vi "pbr-builder.vi"(9 "FLOW in":T3[](array[typedef]), 11 "PBR FLOW in":T2(array[cluster])) -> (1 "PBR FLOW OUT":T2(array[cluster])=[{"Operation"=enum."DELAY SEC", "Param"="5", "uid"=""}, {"Operation"=enum."SENSE", "Param"="5", "uid"=""}, {"Operation"=enum."SENSE", "Param"="a1 > 1.23", "uid"=""}, {"Operation"=enum."SET OUTPUT", "Param"="o1 ON 44", "uid"=""}, {"Operation"=enum."PROC START", "Param"="PROC1", "uid"=""}, {"Operation"=enum."SET OUTPUT", "Param"="PROC1", "uid"=""}], 2 "Err":errorcluster, 3 "FLOW out":T3[](array[typedef]))   [LabVIEW 2024]
uses:
  controls/UiStepBuilder.ctl
  controls/type.step-builder.ctl
  controls/pbr-func-def.ctl
  controls/UiDeviceSensorParams.ctl
  controls/UiDeviceSensorEquality.ctl
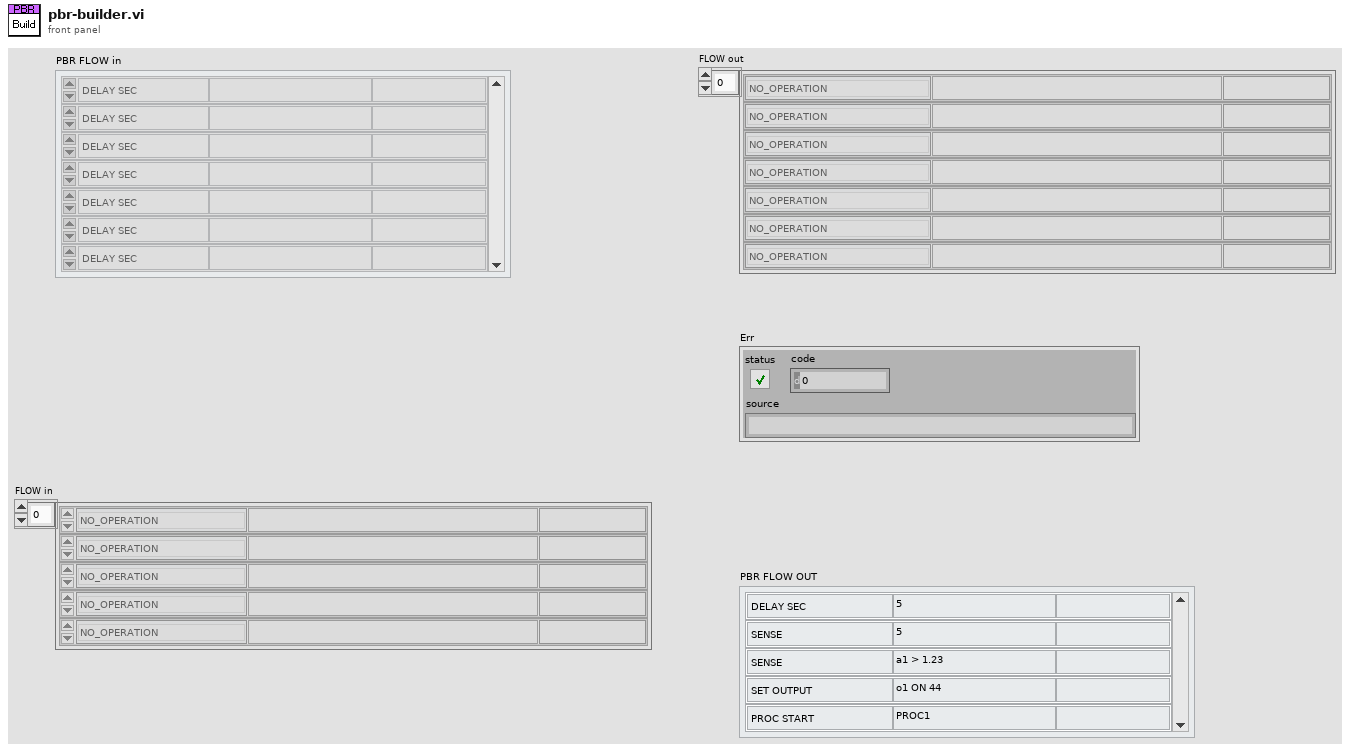
[diagram p1: front panel]
types:
  T1 = typedef "pbr-func-def.ctl" = enum16{"DELAY SEC", "SCHEDULE DAILY", "SENSE", "PROC START", "SET OUTPUT", "FINISH", "JUMP"}
  T2 = cluster{"Operation":T1, "Param":string, "uid":string}[]
  T3 = typedef "UiStepBuilder.ctl" = cluster{"Step Function":T4, "ParamString":string, "Step Label":string}
  T4 = typedef "type.step-builder.ctl" = enum16{"NO_OPERATION", "DELAY-JUMP", "DELAY", "JUMP", "COMPLETE", "SCHEDULER", "SCHEDULER_DAILY", "IRR-CHECK", "UNIT-CHECK", "UNIT-SAMPLE", "UNIT-DOSE", "LOG-REPORT", "LOG-MESSAGE", "IO-READ", "IO-READ-MANY", "IO-WRITE", "IO-COMPARE-OUT", "IO-COMPARE-IN", "PROC-START", "PROC-STOP", "PROC-LOAD", "PROC-IS-COMPLETED", "RECORD-MOVE", "GET-RH", "GET-UV", "GET-WD", "GET-WS", "OCS-CHECK", "OCS-RECORD"}
  T5 = typedef "UiDeviceSensorParams.ctl" = cluster{"Input":string, "Comparison":T6, "Setpoint":dbl}
  T6 = typedef "UiDeviceSensorEquality.ctl" = string
  T7 = cluster{"Operation":T1, "Param":string, "Label":string}
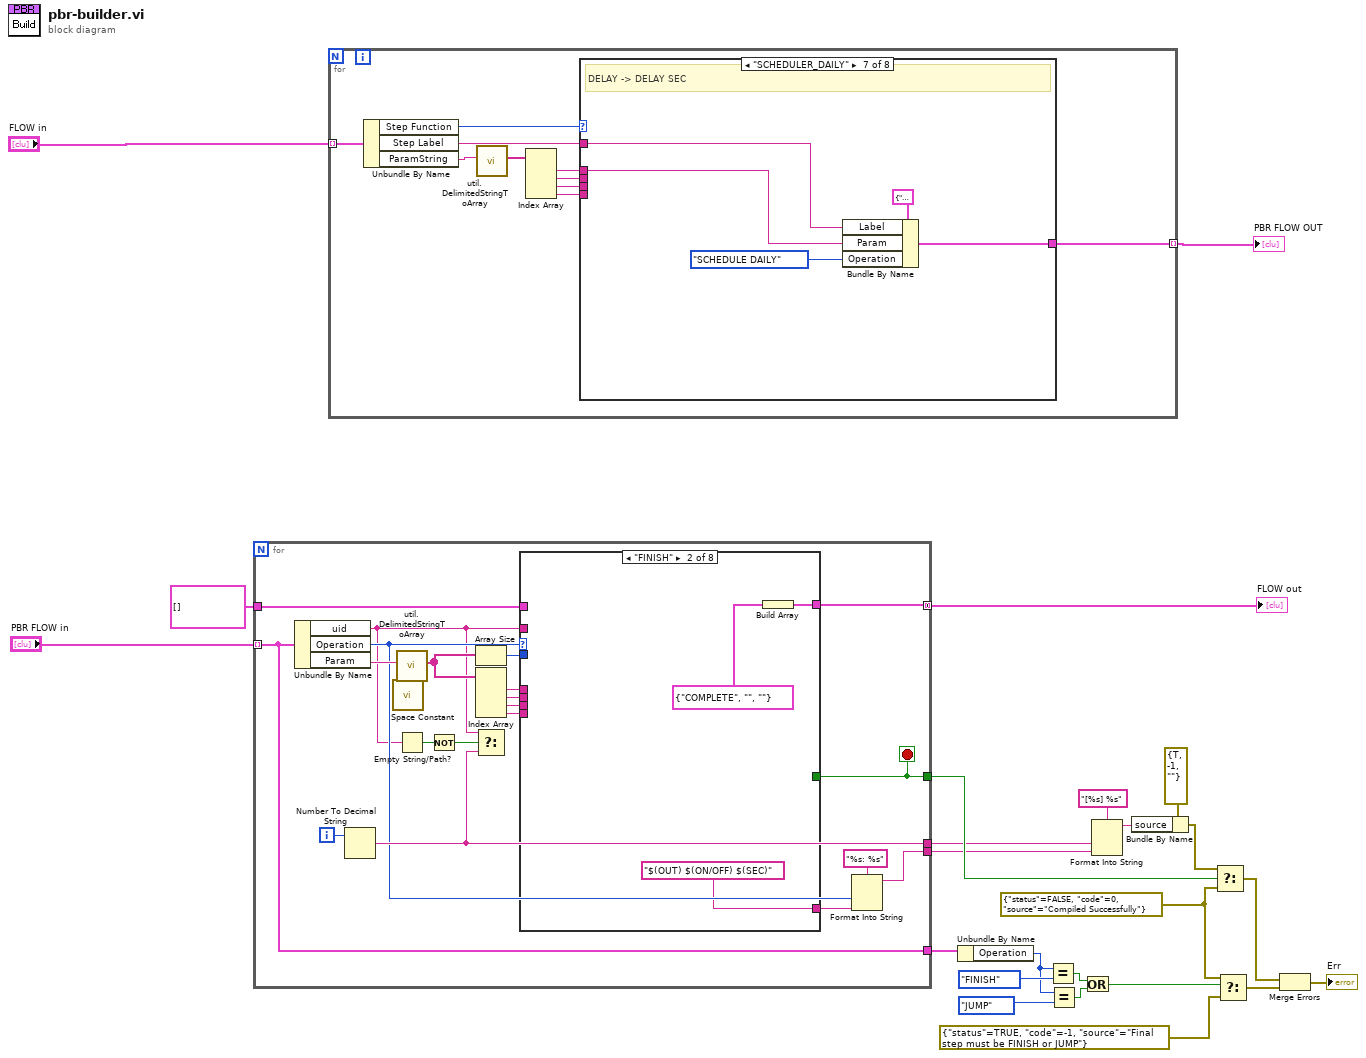
[diagram p0: block diagram]
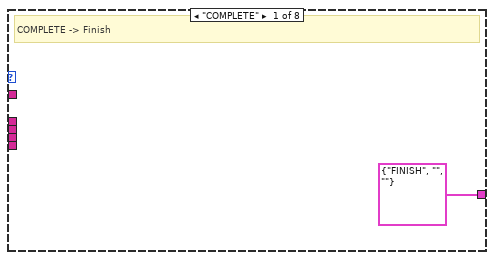
[diagram p2: hidden frame]
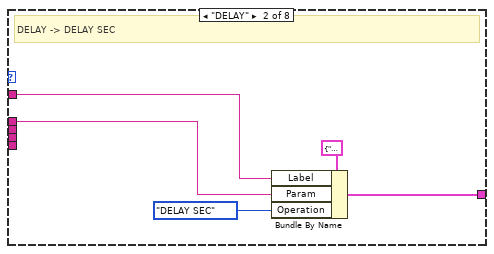
[diagram p3: hidden frame]
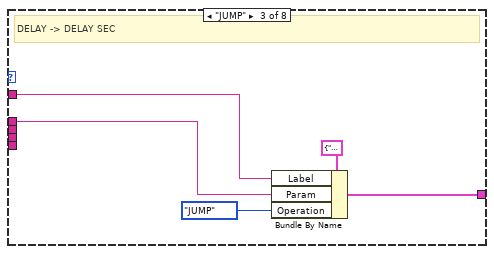
[diagram p4: hidden frame]
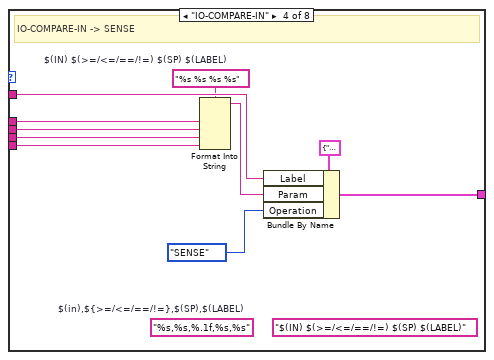
[diagram p5: hidden frame]
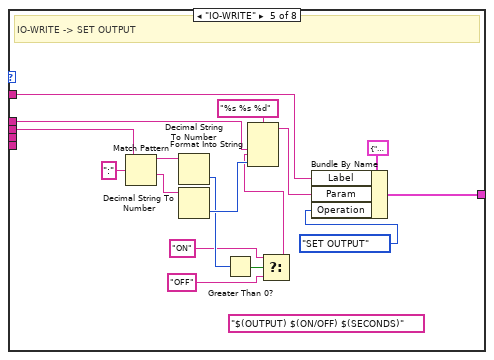
[diagram p6: hidden frame]
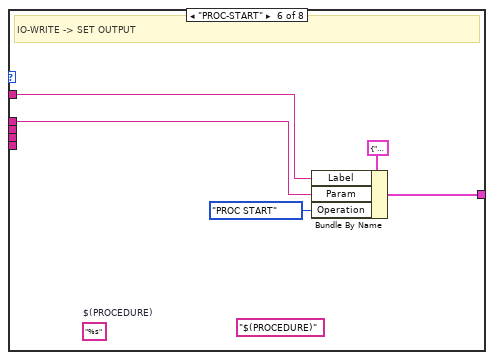
[diagram p7: hidden frame]
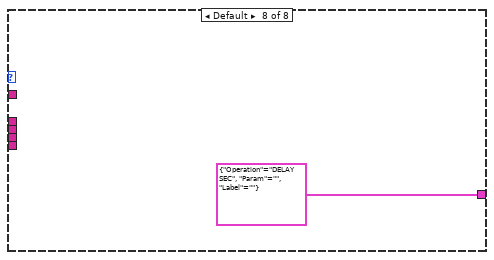
[diagram p8: hidden frame]
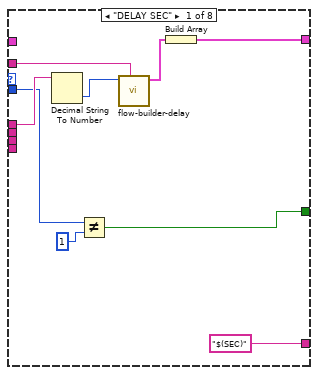
[diagram p9: hidden frame]
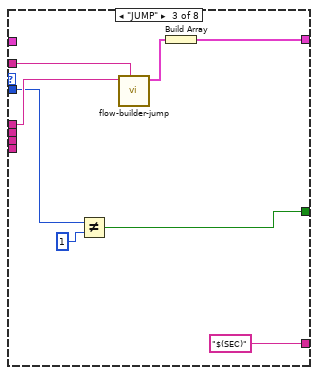
[diagram p10: hidden frame]
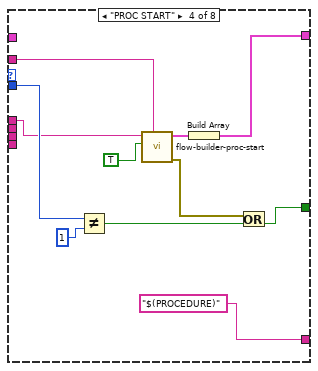
[diagram p11: hidden frame]
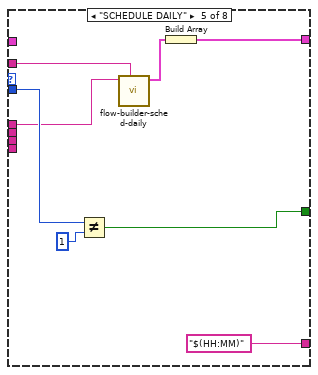
[diagram p12: hidden frame]
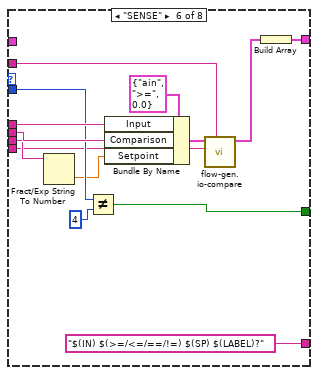
[diagram p13: hidden frame]
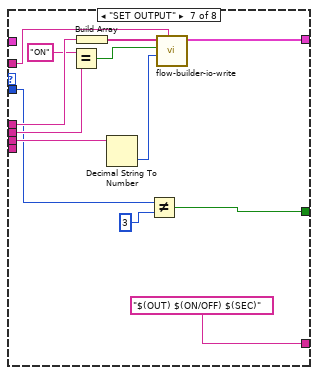
[diagram p14: hidden frame]
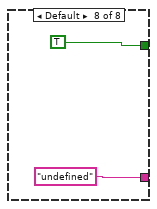
[diagram p15: hidden frame]
diagram:
  w2 = errorcluster {"status"=FALSE, "code"=0, "source"="Compiled Successfully"} ("error constant")
  n1 = for {
    tunnel: "PBR FLOW in" -> [w26] mode=indexing
    tunnel: [w45] -> w13 mode=concatenating
    tunnel: T3[] [] ("UiBuildSteps") -> [w42]
    tunnel: [w35] -> w22
    tunnel: [w34] -> w20
    tunnel: [w28] -> w16
    tunnel: [w26] -> w12
    i -> [w38]
    stop <- w35 stop-if-true
    n2 = Unbundle By Name(w26) -> ("uid"=w25:string, "Operation"=w30:T1, "Param"=w44:string)
    n3 = Number To Decimal String(number=w38) -> (decimal integer string=w34:string)  [unwired: 1 in]
    n4 = call <vilib>:"Space Constant.vi"() -> ("String"=w43:string)
    n5 = call "util.DelimitedStringToArray.vi"("delimiter (,)"=w43, "delimitaed string"=w44) -> ("array out"=w33:string[])  [unwired: 9 in]
    n6 = Empty String/Path?(string/path=w25) -> (empty?=w37:bool)
    n7 = Not(x=w37) -> (.not. x?=w36:bool)
    n8 = Array Size(array=w33) -> (size(s)=w32:i32)
    n9 = Index Array(array=w33) -> (element #1=w41:string, element #2=w40:string, element #3=w39:string, element #4=w27:string)  [unwired: 4 in]
    n10 = Select(t=w25, s=w36, f=w34) -> ()  [unwired: 1 out]
    n11 = case shown="\"FINISH\"" w30 {
      tunnel: w42 -> [_ _ _ _ _ _ _ _]
      tunnel: [w53 w55 w64 w76 w83 w95 w111 _] -> w45
      tunnel: [w47 _ w59 w67 w79 w90 w101 TRUE] -> w35
      tunnel: w41 -> [w52 _ w63 w69 w77 w98 w110 _]
      tunnel: w40 -> [_ _ _ _ _ w97 w108 _]
      tunnel: w25 -> [w50 _ w62 w70 w82 w94 w99 _]
      tunnel: w39 -> [_ _ _ _ _ w96 w104 _]
      tunnel: w32 -> [w48 _ w60 w74 w80 w91 w103 _]
      tunnel: ["$(SEC)" ("y") "$(OUT) $(ON/OFF) $(SEC)" ("y") "$(SEC)" ("y") "$(PROCEDURE)" ("y") "$(HH:MM)" ("y") "$(IN) $(>=/<=/==/!=) $(SP) $(LABEL)?" ("y") "$(OUT) $(ON/OFF) $(SEC)" ("y") "undefined" ("format string")] -> w29
      tunnel: w27 -> [_ _ _ _ _ w85 _ _]
      frame "DELAY SEC" {
        n12 = Decimal String To Number(string=w52) -> (number=w51:i32)  [unwired: 2 in, 1 out]
        n13 = Not Equal?(x=w48, y=1) -> (x != y?=w47:bool)
        n14 = call "flow-builder-delay.vi"("Step Label"=w50, "Delay [s]"=w51) -> ("Step Element"=w54:T3)  [unwired: 9 in]
        n15 = Build Array(w54) -> (w53:T3[])
      }
      frame "FINISH" {
        n16 = Build Array(T3 {"Step Function"=enum."COMPLETE", "ParamString"="", "Step Label"=""} ("FlowModeConstant 2")) -> (w55:T3[])
      }
      frame "JUMP" {
        n17 = Not Equal?(x=w60, y=1) -> (x != y?=w59:bool)
        n18 = call "flow-builder-jump.vi"("Step Label"=w62, "StepPtr"=w63) -> ("Step Element"=w65:T3)  [unwired: 9 in]
        n19 = Build Array(w65) -> (w64:T3[])
      }
      frame "PROC START" {
        n20 = Not Equal?(x=w74, y=1) -> (x != y?=w73:bool)
        n21 = call "flow-builder-proc-start.vi"("Step Label"=w70, "Start(T) / Stop(F)"=TRUE, "Proc Name"=w69) -> ("Error"=w66:errorcluster, "Step Element"=w71:T3)  [unwired: 7 in]
        n22 = Build Array(w71) -> (w76:T3[])
        n23 = Or(x=w66, y=w73) -> (x .or. y?=w67:bool)
      }
      frame "SCHEDULE DAILY" {
        n24 = Not Equal?(x=w80, y=1) -> (x != y?=w79:bool)
        n25 = call "flow-builder-sched-daily.vi"("Step Label"=w82, "time (HH:MM)"=w77) -> ("Step Element"=w84:T3)  [unwired: 9 in]
        n26 = Build Array(w84) -> (w83:T3[])
      }
      frame "SENSE" {
        n27 = Fract/Exp String To Number(string=w96) -> (number=w89:dbl)  [unwired: 3 in, 1 out]
        n28 = Not Equal?(x=w91, y=4) -> (x != y?=w90:bool)
        n29 = Bundle By Name(cluster=T5 {"Input"="ain", "Comparison"=">=", "Setpoint"=0.0} ("Device Sensor Params"), "Input"=w98, "Comparison"=w97, "Setpoint"=w89) -> (w87:T5)
        n30 = call "flow-gen.io-compare.vi"("Step Label"=w94, "stepPointer (False Cond.)"=w85, "Device Sensor Params"=w87) -> ("Step out"=w86:T3)  [unwired: 8 in]
        n31 = Build Array(w86) -> (w95:T3[])
      }
      frame "SET OUTPUT" {
        n32 = Equal?(x=w108, y="ON") -> (x = y?=w106:bool)
        n33 = Build Array(w110) -> (w109:string[])
        n34 = Decimal String To Number(string=w104) -> (number=w105:i32)  [unwired: 2 in, 1 out]
        n35 = Not Equal?(x=w103, y=3) -> (x != y?=w101:bool)
        n36 = call "flow-builder-io-write.vi"("Step Name"=w99, "Digital Timeout"=w105, "Value in"=w106, "Dout+AUX"=w109) -> ("Flow out"=w111:T3[])  [unwired: 7 in]
      }
      frame Default {
      }
    }
    n37 = Format Into String(format string="%s: %s", w30, w29) -> (resulting string=w28:string)  [unwired: 2 in, 1 out]
  }
  "FLOW out" <- w13
  n38 = for {
    tunnel: "FLOW in" -> [w123] mode=indexing
    tunnel: [w121] -> w15 mode=indexing
    n39 = Unbundle By Name(w123) -> ("Step Function"=w122:T4, "Step Label"=w120:string, "ParamString"=w119:string)
    n40 = call "util.DelimitedStringToArray.vi"("delimitaed string"=w119) -> ("array out"=w118:string[])  [unwired: 10 in]
    n41 = Index Array(array=w118) -> (element #1=w117:string, element #2=w116:string, element #3=w115:string, element #4=w114:string)  [unwired: 4 in]
    n42 = case shown="\"SCHEDULER_DAILY\"" w122 {
      tunnel: [T7 {"Operation"=enum."FINISH", "Param"="", "Label"=""} w129 w134 w144 w161 w166 w171 T7 {"Operation"=enum."DELAY SEC", "Param"="", "Label"=""}] -> w121
      tunnel: w120 -> [_ w128 w133 w143 w160 w165 w170 _]
      tunnel: w117 -> [_ w125 w130 w138 w146 w163 w167 _]
      tunnel: w116 -> [_ _ _ w137 w145 _ _ _]
      tunnel: w115 -> [_ _ _ w136 _ _ _ _]
      tunnel: w114 -> [_ _ _ w135 _ _ _ _]
      frame "COMPLETE" {
        # "COMPLETE -> Finish"
      }
      frame "DELAY" {
        # "DELAY -> DELAY SEC"
        n43 = Bundle By Name(cluster=T7 {"Operation"=enum."DELAY SEC", "Param"="", "Label"=""}, "Label"=w128, "Param"=w125, "Operation"=pbr-func-def."DELAY SEC") -> (w129:T7)
      }
      frame "JUMP" {
        # "DELAY -> DELAY SEC"
        n44 = Bundle By Name(cluster=T7 {"Operation"=enum."DELAY SEC", "Param"="", "Label"=""}, "Label"=w133, "Param"=w130, "Operation"=pbr-func-def."JUMP") -> (w134:T7)
      }
      frame "IO-COMPARE-IN" {
        (unwired) "%s,%s,%.1f,%s,%s"  # $(in),${>=/<=/==/!=},$(SP),$(LABEL)
        (unwired) "$(IN) $(>=/<=/==/!=) $(SP) $(LABEL)" ("y")
        w140 = "%s %s %s %s"  # $(IN) $(>=/<=/==/!=) $(SP) $(LABEL)
        # "IO-COMPARE-IN -> SENSE"
        n45 = Format Into String(format string=w140, w138, w137, w136, w135) -> (resulting string=w139:string)  [unwired: 2 in, 1 out]
        n46 = Bundle By Name(cluster=T7 {"Operation"=enum."DELAY SEC", "Param"="", "Label"=""}, "Label"=w143, "Param"=w139, "Operation"=pbr-func-def."SENSE") -> (w144:T7)
      }
      frame "IO-WRITE" {
        (unwired) "$(OUTPUT) $(ON/OFF) $(SECONDS)" ("y")
        # "IO-WRITE -> SET OUTPUT"
        n47 = Match Pattern(string=w145, regular expression=":") -> (before substring=w154:string, after substring=w153:string)  [unwired: 1 in, 2 out]
        n48 = Decimal String To Number(string=w154) -> (number=w151:i32)  [unwired: 2 in, 1 out]
        n49 = Decimal String To Number(string=w153) -> (number=w152:i32)  [unwired: 2 in, 1 out]
        n50 = Greater Than 0?(x=w151) -> (x > 0?=w150:bool)
        n51 = Select(t="ON" ("format string"), s=w150, f="OFF" ("format string")) -> (s? t:f=w147:string)
        n52 = Format Into String(format string="%s %s %d", w146, w147, w152) -> (resulting string=w156:string)  [unwired: 2 in, 1 out]
        n53 = Bundle By Name(cluster=T7 {"Operation"=enum."DELAY SEC", "Param"="", "Label"=""}, "Label"=w160, "Param"=w156, "Operation"=pbr-func-def."SET OUTPUT") -> (w161:T7)
      }
      frame "PROC-START" {
        (unwired) "%s"  # $(PROCEDURE)
        (unwired) "$(PROCEDURE)" ("y")
        # "IO-WRITE -> SET OUTPUT"
        n54 = Bundle By Name(cluster=T7 {"Operation"=enum."DELAY SEC", "Param"="", "Label"=""}, "Label"=w165, "Param"=w163, "Operation"=pbr-func-def."PROC START") -> (w166:T7)
      }
      frame "SCHEDULER_DAILY" {
        # "DELAY -> DELAY SEC"
        n55 = Bundle By Name(cluster=T7 {"Operation"=enum."DELAY SEC", "Param"="", "Label"=""}, "Label"=w170, "Param"=w167, "Operation"=pbr-func-def."SCHEDULE DAILY") -> (w171:T7)
      }
      frame Default {
      }
    }
  }
  "PBR FLOW OUT" <- w15
  n56 = Unbundle By Name(w12) -> ("Operation"=w10:T1)
  n57 = Equal?(x=w10, y=pbr-func-def."FINISH" ("Operation")) -> (x = y?=w8:bool)
  n58 = Equal?(x=w10, y=pbr-func-def."JUMP" ("Operation")) -> (x = y?=w7:bool)
  n59 = Or(x=w8, y=w7) -> (x .or. y?=w3:bool)
  n60 = Format Into String(format string="[%s] %s", w20, w16) -> (resulting string=w18:string)  [unwired: 2 in, 1 out]
  n61 = Bundle By Name(cluster=errorcluster {"status"=TRUE, "code"=-1, "source"=""} ("error constant"), "source"=w18) -> (w17:errorcluster)
  n62 = Select(t=w17, s=w22, f=w2) -> (s? t:f=w6:errorcluster)
  n63 = Select(t=w2, s=w3, f=errorcluster {"status"=TRUE, "code"=-1, "source"="Final step must be FINISH or JUMP"} ("error constant")) -> (s? t:f=w1:errorcluster)
  n64 = Merge Errors(w6, w1) -> (→"Err":errorcluster)
